vi "writeToXML.vi"(8 "error in (no error)":errorcluster, 10 "ClassLabel":string, 11 "POriginCommands in":refnum<class "POriginCommands.lvclass">) -> (0 "error out":errorcluster, 2 "XML out":string, 3 "POriginCommands out":refnum<class "POriginCommands.lvclass">)   [LabVIEW 2022 SP3, in "TCSDataDefinitions.lvlib" / "TCSCommand.lvlib" / "POriginCommands.lvlib" / "POriginCommands.lvclass"]
uses:
  POriginCommands.lvclass
  TCSTcsCommand/TCSTcsCommand.lvclass
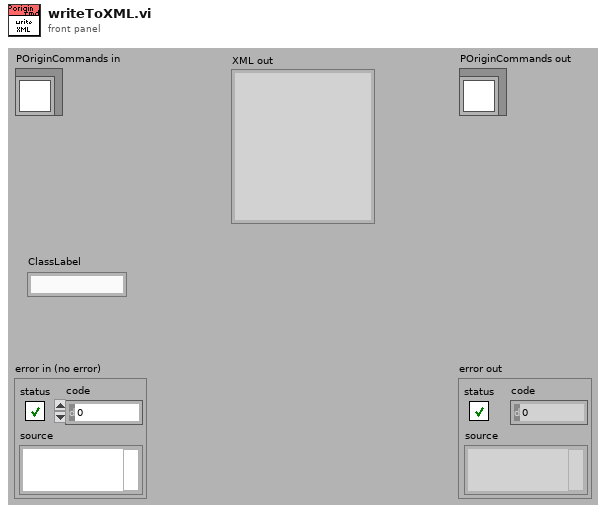
[diagram p1: front panel]
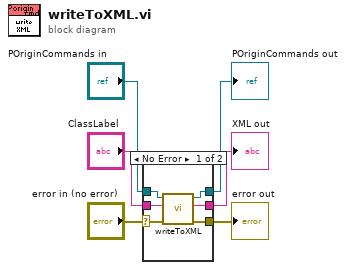
[diagram p0: block diagram]
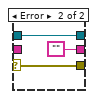
[diagram p2: hidden frame]
diagram:
  n1 = case shown="No Error" "error in (no error)" {
    selector: "error in (no error)" -> [w11 w15]
    tunnel: [w10 w15] -> w5
    tunnel: [w8 w14] -> w3
    tunnel: "POriginCommands in" -> [w9 w14]
    tunnel: "ClassLabel" -> [w12 _]
    tunnel: [w7 ""] -> w1
    frame No Error {
      n2 = call-parent "writeToXML.vi"("error in (no error)"=w11, "ClassLabel"=w12, "TCSTcsCommand in"=w9) -> ("error out"=w10:errorcluster, "XML out"=w7:string, "TCSTcsCommand out"=w8:refnum<class "POriginCommands.lvclass">)  [unwired: 6 in]
    }
    frame Error {
    }
  }
  "error out" <- w5
  "POriginCommands out" <- w3
  "XML out" <- w1
